vi "_backward multiply grad.vi"(7 "In":refnum<class "Value.lvclass">, 8 "error in":errorcluster, 10 "out grad":T1, 11 "variant":variant) -> (0 "error out":errorcluster, 3 "out":variant)   [LabVIEW 2023, in "LabGRAD.lvlib" / "Value.lvclass"]
uses:
  Value.lvclass
  Value.lvclass/Value.ctl
  UiObjects/numeric value control.ctl
  UiObjects/UiObjects.lvclass
panel:
  out "Out":refnum<class "Value.lvclass">
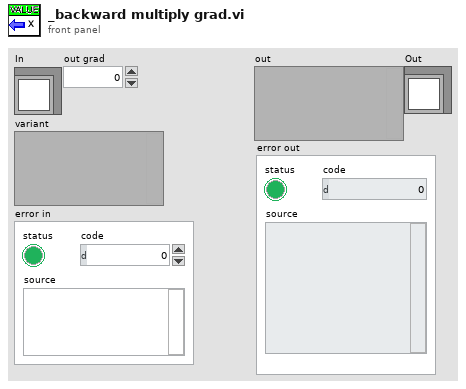
[diagram p1: front panel]
types:
  T1 = typedef "UiObjects.lvlib/UiObjects.lvclass/numeric value control.ctl" = dbl
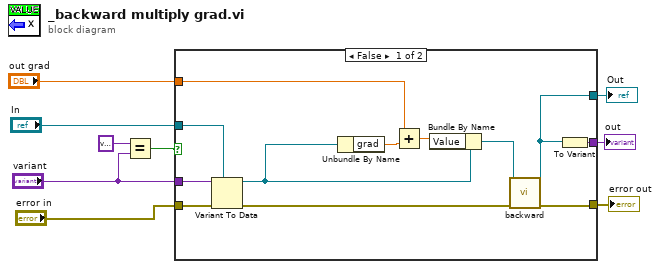
[diagram p0: block diagram]
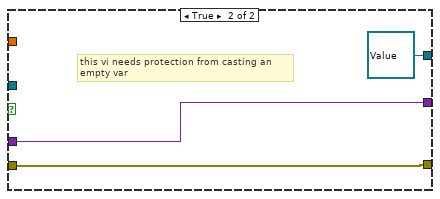
[diagram p2: hidden frame]
diagram:
  n1 = Equal?(x=variant, y="variant") -> (x = y?=w2:bool)
  n2 = case shown="False" w2 {
    tunnel: "variant" -> [w20 w23]
    tunnel: "In" -> [w19 _]
    tunnel: "out grad" -> [w17 _]
    tunnel: [w15 w23] -> w7
    tunnel: "error in" -> [w14 w24]
    tunnel: [w12 w24] -> w5
    tunnel: [w10 refnum<class "Value.lvclass"> refnum ("Out")] -> w1
    frame False {
      n3 = Variant To Data(error in=w14, type=w19, Variant=w20) -> (data=w16:refnum<class "Value.lvclass">, error out=w13:errorcluster)
      n4 = Unbundle By Name(w16) -> ("grad"=w18:T1)
      n5 = Add(x=w17, y=w18) -> (x+y=w21:T1)
      n6 = Bundle By Name(cluster=w16, "Value"=w21) -> (w11:refnum<class "Value.lvclass">)
      n7 = call "backward.vi"("i"=w13, "In"=w11) -> ("error out"=w12:errorcluster, "Out"=w10:refnum<class "Value.lvclass">)  [unwired: 8 in]
      n8 = To Variant(anything=w10) -> (Variant=w15:variant)
    }
    frame True {
      # "this vi needs protection from casting an \nempty var"
    }
  }
  "out" <- w7
  "error out" <- w5
  "Out" <- w1
